vi "Create DC Waveforms.vi"(8 "error in (no error)":errorcluster, 11 "Generator in":refnum<class "Generator.lvclass">) -> (0 "Error out":errorcluster, 2 "Waveforms out":waveform(dbl)[](array[waveform]), 3 "Generator out":refnum<class "Generator.lvclass">)   [LabVIEW 2019, in "Generator.lvclass"]
uses:
  Generator.lvclass
  Generator.lvclass/Generator.ctl
  63fde90b-2159-4c8a-ab22-01bff570a163.vi
  2391b7ef-af54-4c2f-83c4-48dc17038844.vi
panel:
  out "reset wfm":bool
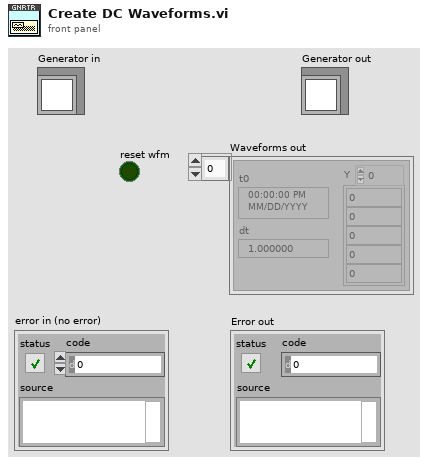
[diagram p1: front panel]
types:
  T1 = typedef "Generator.lvclass/AO.Channel--Cluster--Array.ctl" = T2[]
  T2 = typedef "Generator.lvclass/AO.Channel--Cluster.ctl" = cluster{"Enable?":bool, "Channel":i32, "Amplitude":dbl, "Offset":dbl, "Frequency":dbl, "Phase":dbl, "Function":T3, "Sweeping?":bool, "Limit AC?":bool, "Limit DC?":bool, "Duty Cycle?":bool, "Duty Cycle":dbl}
  T3 = typedef "Generator.lvclass/AO.Channel.Function--Enum.ctl" = enum16{"sine", "square", "triangle", "saw"}
  T4 = typedef "Generator.lvclass/Sampling--Cluster.ctl" = cluster{"Fs":dbl, "#s":dbl}
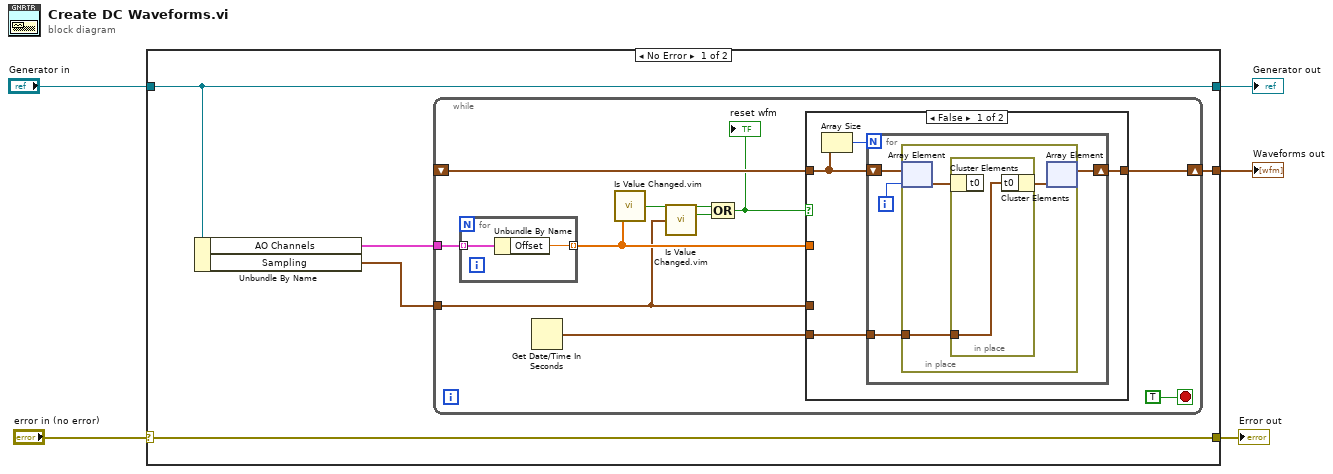
[diagram p0: block diagram]
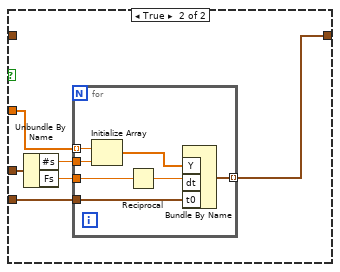
[diagram p2: hidden frame]
diagram:
  n1 = case shown="No Error" "error in (no error)" {
    selector: "error in (no error)" -> [w9 w49]
    tunnel: [w10 _] -> w5
    tunnel: [w9 w49] -> w3
    tunnel: [w7 w48] -> w2
    tunnel: "Generator in" -> [w7 w48]
    frame No Error {
      n2 = Unbundle By Name(w7) -> ("AO Channels"=w8:T1, "Sampling"=w6:T4)
      n3 = while {
        tunnel: w8 -> [w18]
        tunnel: w6 -> [w11]
        shift-right: [w20] -> w10
        shift-left: _ -> [w16]
        stop <- TRUE stop-if-true
        n4 = for {
          tunnel: w18 -> [w47] mode=indexing
          tunnel: [w46] -> w12 mode=indexing
          n5 = Unbundle By Name(w47) -> ("Offset"=w46:dbl)
        }
        n6 = Get Date/Time In Seconds() -> (seconds since 1Jan1904=w19:timestamp)
        n7 = call "Is Value Changed.vim"("value"=w12) -> ("changed or first call?"=w13:bool)
        n8 = call "Is Value Changed.vim"("value"=w11) -> ("changed or first call?"=w14:bool)
        n9 = Compound Arithmetic op=OR(w13, w14) -> (w15:bool)
        "reset wfm" <- w15
        n10 = case shown="False" w15 {
          tunnel: [w21 w38] -> w20
          tunnel: w19 -> [w22 w37]
          tunnel: w12 -> [_ w34]
          tunnel: w11 -> [_ w33]
          tunnel: w16 -> [w23 _]
          frame False {
            n11 = Array Size(array=w23) -> (size(s)=w24:i32)
            n12 = for {
              N: w24 -> [_]
              shift-right: [w27] -> w21
              shift-left: w23 -> [w28]
              tunnel: w22 -> [w25]
              i -> [w26]
              n13 = in-place {
                in-place-border: w25 -> [w30]
                n14 = in-place-array #1(w28, w26) -> (w31:waveform(dbl))
                n15 = in-place {
                  in-place-border: w30 -> [w32]
                  n16 = in-place-cluster #2(w31) -> ()  [unwired: 1 out]
                  n17 = in-place-cluster #2("t0"=w32) -> (w29:waveform(dbl))
                }
                n18 = in-place-array #1(w29) -> (w27:waveform(dbl)[])  [unwired: 1 out]
              }
            }
          }
          frame True {
            n19 = Unbundle By Name(w33) -> ("#s"=w35:dbl, "Fs"=w36:dbl)
            n20 = for {
              tunnel: w35 -> [w44]
              tunnel: w34 -> [w45] mode=indexing
              tunnel: w36 -> [w42]
              tunnel: w37 -> [w40]
              tunnel: [w39] -> w38 mode=indexing
              n21 = Initialize Array(w45, w44) -> (w41:dbl[])
              n22 = Reciprocal(x=w42) -> (1/x=w43:dbl)
              n23 = Bundle By Name("Y"=w41, "dt"=w43, "t0"=w40) -> (w39:waveform(dbl))  [unwired: 1 in]
            }
          }
        }
      }
    }
    frame Error {
    }
  }
  "Waveforms out" <- w5
  "Error out" <- w3
  "Generator out" <- w2
